vi "GSM Modify Standard.vi"(0 "VISA Resource Name":refnum<visa-resource-name>, 1 "Diff Encode  (T:ON)":bool=TRUE, 2 "Filter BbT (0.30)":dbl=0.3 format="%.2f", 3 "Bit Rate (270.833)":dbl=270.833 format="%.3f", 5 "Phase Polarity (T:NORMAL)":bool=TRUE, 7 "Burst Rise Time (4.220)":dbl=4.22 format="%.3f", 9 "Burst Rise Delay (0)":dbl format="%.3f", 11 "error in (no error)":errorcluster {"code" format="%.0x"}, 12 "Burst Fall Time (3.44)":dbl=3.44 format="%.3f", 13 "Burst Fall Delay (4.38)":dbl=4.38 format="%.3f") -> (4 "VISA Resource Name Out":refnum<visa-resource-name>, 15 "error out":errorcluster {"code" format="%.0x"})   [LabVIEW 2012, in "Agilent ESG Series.lvlib"]
doc: "This VI is used to configure the \"Modify Standard\" parameters."
uses:
  <instrlib>/Agilent ESG Series/Agilent ESG Series.lvlib
panel:
  # "NORMAL"
  # "INVERT"
  # "ON"
  # "OFF"
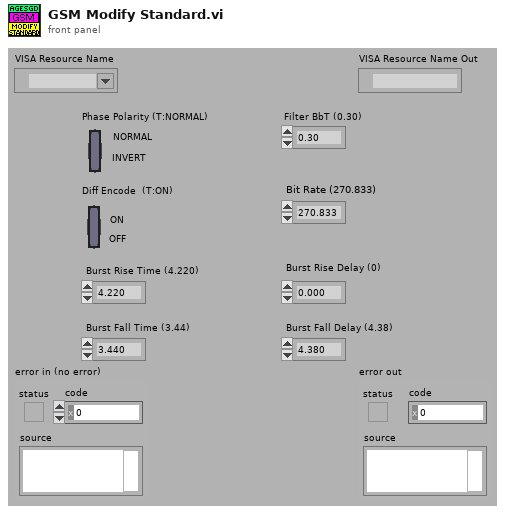
[diagram p1: front panel]
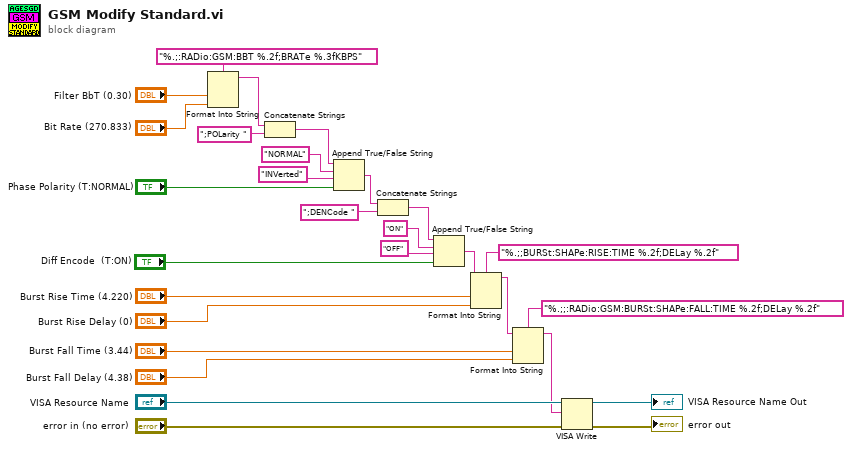
[diagram p0: block diagram]
diagram:
  n1 = Format Into String(format string="%.;:RADio:GSM:BBT %.2f;BRATe %.3fKBPS", "Filter BbT (0.30)", "Bit Rate (270.833)") -> (resulting string=w17:string)  [unwired: 2 in, 1 out]
  n2 = Concatenate Strings(w17, ";POLarity ") -> (w21:string)
  n3 = Append True/False String(1:"Phase Polarity (T:NORMAL)", 2:"INVerted" ("false string"), 3:"NORMAL" ("true string"), 4:w21) -> (0:w2:string)
  n4 = Concatenate Strings(w2, ";DENCode ") -> (w4:string)
  n5 = Append True/False String(1:"Diff Encode  (T:ON)", 2:"OFF" ("false string"), 3:"ON" ("true string"), 4:w4) -> (0:w1:string)
  n6 = Format Into String(format string="%.;;BURSt:SHAPe:RISE:TIME %.2f;DELay %.2f", initial string=w1, "Burst Rise Time (4.220)", "Burst Rise Delay (0)") -> (resulting string=w12:string)  [unwired: 1 in, 1 out]
  n7 = Format Into String(format string="%.;;:RADio:GSM:BURSt:SHAPe:FALL:TIME %.2f;DELay %.2f", initial string=w12, "Burst Fall Time (3.44)", "Burst Fall Delay (4.38)") -> (resulting string=w8:string)  [unwired: 1 in, 1 out]
  n8 = VISA Write(VISA resource name="VISA Resource Name", write buffer=w8, error in (no error)="error in (no error)") -> (VISA resource name out=→"VISA Resource Name Out":refnum<visa-resource-name>, error out=→"error out":errorcluster)  [unwired: 1 out]
